vi "isHomed.vi"(5 "Device in":refnum<k24>) -> (2 "Device out":refnum<k24>)   [LabVIEW 2014]
doc: "André Romero - 2017\nandretec@ifsc.usp.br"
uses:
  C:/UserLabs/Andre/LabView2014-32bits/kinesisTec/Kinesis/Thorlabs.MotionControl.TCube.DCServoCLI.dll
  Kinesis/Thorlabs.MotionControl.TCube.DCServoCLI.dll
  C:/UserLabs/Andre/LabView2014-32bits/kinesisTec/Kinesis/Thorlabs.MotionControl.GenericMotorCLI.dll
  Kinesis/Thorlabs.MotionControl.GenericMotorCLI.dll
  motorsGlobalVar.vi
panel:
  out "IsHomed":bool
  out "SerialNumber":u32
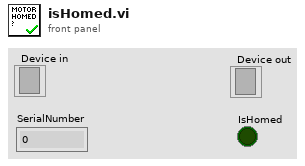
[diagram p1: front panel]
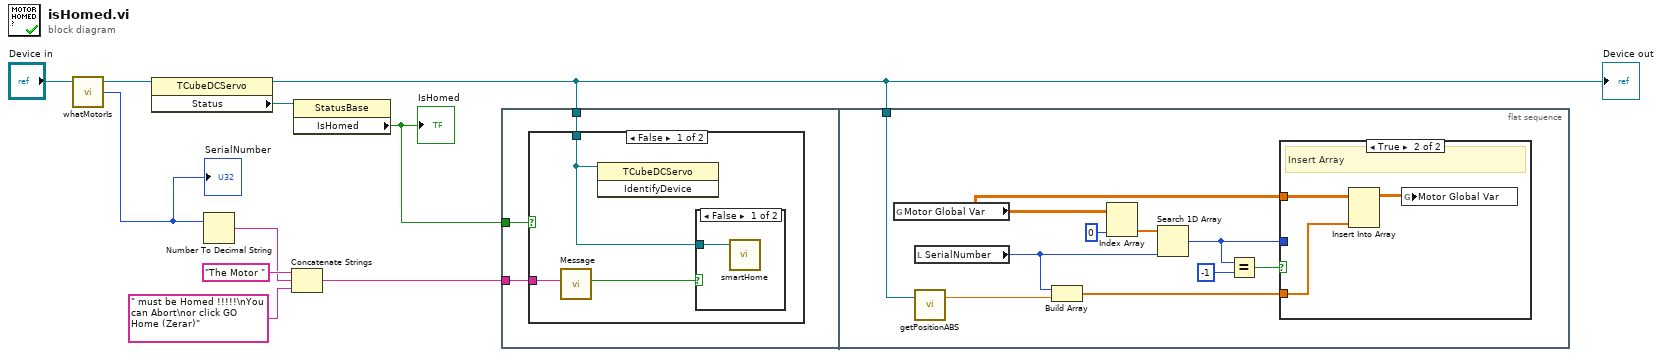
[diagram p0: block diagram]
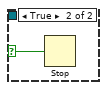
[diagram p2: hidden frame]
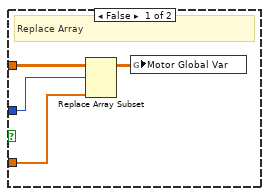
[diagram p4: hidden frame]
diagram:
  n1 = call "whatMotorIs.vi"("Device in"="Device in") -> ("SerialNumber"=w8:u32, "Device out"=w2:refnum<k24>)  [unwired: 3 in]
  "SerialNumber" <- w8
  n2 = property class="TCubeDCServo"(reference=w2) -> (reference out=w1:refnum<k24>, "Status"=w9:refnum<k24>)  [unwired: 1 in, 1 out]
  "Device out" <- w1
  n3 = Number To Decimal String(number=w8) -> (decimal integer string=w6:string)  [unwired: 1 in]
  n4 = Concatenate Strings("The Motor ", w6, " must be Homed !!!!!\nYou can Abort\nor click GO Home (Zerar)" ("string")) -> (w4:string)
  n5 = property class="StatusBase"(reference=w9) -> ("IsHomed"=w10:bool)  [unwired: 1 in, 2 out]
  "IsHomed" <- w10
  n6 = flat-sequence {
    tunnel: w10 -> [w13]
    tunnel: w4 -> [w12]
    tunnel: w1 -> [w11]
    tunnel: w1 -> [w22]
    frame #0 {
      n7 = case shown="False" w13 {
        tunnel: w12 -> [w16 _]
        tunnel: w11 -> [w14 _]
        frame False {
          n8 = call "Message"("Message"=w16) -> ("Abort"=w15:bool)  [unwired: 9 in, 1 out]
          n9 = invoke class="TCubeDCServo" method="IdentifyDevice"(reference=w14) -> ()  [unwired: 2 in, 3 out]
          n10 = case shown="False" w15 {
            selector: w15 -> [_ w18]
            tunnel: w14 -> [w17 _]
            frame False {
              n11 = call "smartHome.vi"("Device in"=w17) -> ()  [unwired: 4 in, 1 out]
            }
            frame True {
              n12 = Stop(stop? (T)=w18) -> ()
            }
          }
        }
        frame True {
        }
      }
    }
    frame #1 {
      n13 = global read "motorsGlobalVar.vi" "Motor Global Var"() -> (w23:dbl[][])
      n14 = local read "SerialNumber"() -> (w21:u32)
      n15 = call "getPositionABS.vi"("Device"=w22) -> ("GetPOS"=w20:dbl)  [unwired: 2 in]
      n16 = Build Array(w21, w20) -> (w19:dbl[])
      n17 = Index Array(array=w23, index (col)=0 ("disabled index (col)")) -> (element=w27:dbl[])  [unwired: 1 in]
      n18 = Search 1D Array(1D array=w27, element=w21) -> (index of element=w24:i32)  [unwired: 1 in]
      n19 = Equal?(x=w24, y=-1) -> (x = y?=w25:bool)
      n20 = case shown="True" w25 {
        tunnel: w24 -> [w31 _]
        tunnel: w23 -> [w32 w35]
        tunnel: w19 -> [w30 w34]
        frame False {
          # "Replace Array"
          n21 = Replace Array Subset(array=w32, new element=w30, index (row)=w31) -> (w29:dbl[][])  [unwired: 1 in]
          n22 = global write "motorsGlobalVar.vi" "Motor Global Var"(w29) -> ()
        }
        frame True {
          # "Insert Array"
          n23 = Insert Into Array(array=w35, new element=w34) -> (w33:dbl[][])  [unwired: 2 in]
          n24 = global write "motorsGlobalVar.vi" "Motor Global Var"(w33) -> ()
        }
      }
    }
  }
